vi "AskForConnectedMonos.vi"(7 "DiscoverDevices in":T1, 8 "error in (no error)":errorcluster, 10 "timeout for receiving data [ms]":i32=5000, 11 "Communicator in":refnum<class "Communicator.lvclass">) -> (0 "error out":errorcluster, 2 "DiscoverDevices out":T1, 3 "Communicator out":refnum<class "Communicator.lvclass">)   [LabVIEW 2023, in "horiba.lvlib" / "DeviceManager.lvlib"]
uses:
  DeviceManager.lvlib
  DiscoverDevices (Reply Payload)--cluster.ctl
  Communicator/Communicator.lvclass
  Mono/Monochromator.lvclass
  GenericDevice/GenericDevice.lvclass
  CCD/CCD.lvclass
  SCD/SCD.lvclass
panel:
  # "Connector Pane"
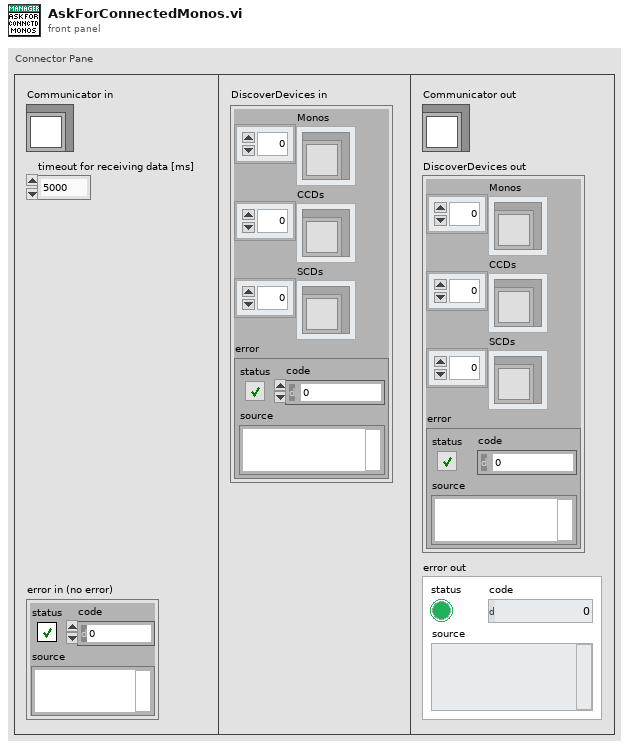
[diagram p1: front panel]
types:
  T1 = typedef "horiba.lvlib/DeviceManager.lvlib/DiscoverDevices (Reply Payload)--cluster.ctl" = cluster{"Monos":refnum<class "Monochromator.lvclass">[], "CCDs":refnum<class "CCD.lvclass">[], "SCDs":refnum<class "SCD.lvclass">[], "error":errorcluster}
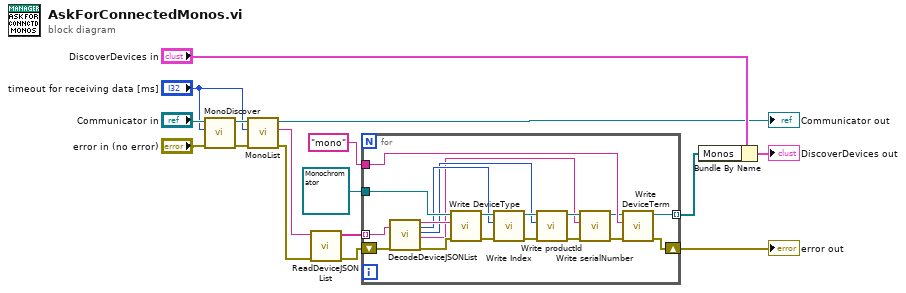
[diagram p0: block diagram]
diagram:
  n1 = call "MonoDiscover.vi"("error in (no error)"="error in (no error)", "Delay between send and receive [ms]"="timeout for receiving data [ms]", "Communicator in"="Communicator in") -> ("error out"=w2:errorcluster, "Communicator out"=w10:refnum<class "Communicator.lvclass">)  [unwired: 5 in, 2 out]
  n2 = call "MonoList.vi"("error in (no error)"=w2, "Delay between send and receive [ms]"="timeout for receiving data [ms]", "Communicator in"=w10) -> ("error out"=w5:errorcluster, "results-JSON"=w4:string, "Communicator out"=→"Communicator out":refnum<class "Communicator.lvclass">)  [unwired: 5 in, 1 out]
  n3 = call "ReadDeviceJSONList.vi"("error in"=w5, "JSON"=w4) -> ("error out"=w12:errorcluster, "table of devices"=w13:string[])  [unwired: 8 in]
  n4 = for {
    tunnel: w13 -> [w32] mode=indexing
    shift-right: [w28] -> w14
    shift-left: w12 -> [w31]
    tunnel: [w29] -> w1 mode=indexing
    tunnel: "mono" -> [w30]
    tunnel: refnum<class "Monochromator.lvclass"> refnum ("Monochromator.lvclass") -> [w21]
    n5 = call "DecodeDeviceJSONList.vi"("JSON"=w32, "error in"=w31) -> ("deviceType"=w20:string, "index"=w19:i32, "productId"=w18:i32, "serialNumber"=w17:string, "error out"=w34:errorcluster)  [unwired: 12 in, 1 out]
    n6 = call-dynamic "Write DeviceType.vi"("error in (no error)"=w34, "device type"=w20, "Monochromator in"=w21) -> ("error out"=w33:errorcluster, "Monochromator out"=w35:refnum<class "Monochromator.lvclass">)  [unwired: 7 in]
    n7 = call-dynamic "Write Index.vi"("error in (no error)"=w33, "Index"=w19, "Monochromator in"=w35) -> ("error out"=w25:errorcluster, "Monochromator out"=w27:refnum<class "Monochromator.lvclass">)  [unwired: 7 in]
    n8 = call-dynamic "Write productId.vi"("error in (no error)"=w25, "productId"=w18, "Monochromator in"=w27) -> ("error out"=w24:errorcluster, "Monochromator out"=w26:refnum<class "Monochromator.lvclass">)  [unwired: 7 in]
    n9 = call-dynamic "Write serialNumber.vi"("error in (no error)"=w24, "serialNumber"=w17, "Monochromator in"=w26) -> ("error out"=w22:errorcluster, "Monochromator out"=w23:refnum<class "Monochromator.lvclass">)  [unwired: 7 in]
    n10 = call-dynamic "Write DeviceTerm.vi"("error in (no error)"=w22, "deviceTerm"=w30, "Monochromator in"=w23) -> ("error out"=w28:errorcluster, "Monochromator out"=w29:refnum<class "Monochromator.lvclass">)  [unwired: 7 in]
  }
  "error out" <- w14
  n11 = Bundle By Name(cluster="DiscoverDevices in", "Monos"=w1) -> (→"DiscoverDevices out":T1)
